vi "Read Regions.vi"(8 "error in (no error)":errorcluster, 11 "SOL Camera in":refnum<class "PL SOL Instruments Camera.lvclass">) -> (0 "error out":errorcluster, 2 "regions":T1(array[cluster]), 3 "SOL Camera out":refnum<class "PL SOL Instruments Camera.lvclass">)   [LabVIEW 2015, in "PL SOL Instruments Camera.lvclass"]
doc: "Reads acquisition regions."
uses:
  PL SOL Instruments Camera.lvclass
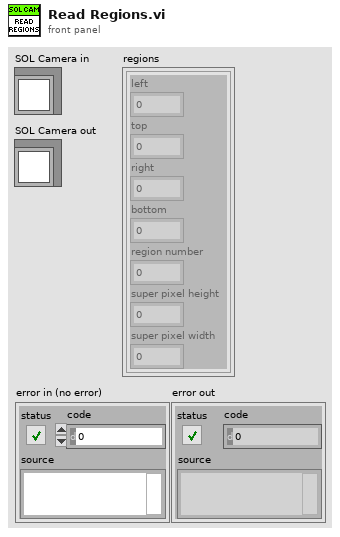
[diagram p1: front panel]
types:
  T1 = cluster{"left":u16, "top":u16, "right":u16, "bottom":u16, "region number":u16, "super pixel height":u16, "super pixel width":u16}[]
  T2 = cluster{"wLeft":u16, "wTop":u16, "wRight":u16, "wBottom":u16, "wRegionNumber":u16, "wSUPixelHeight":u16, "wSUPixelWidth":u16}[]
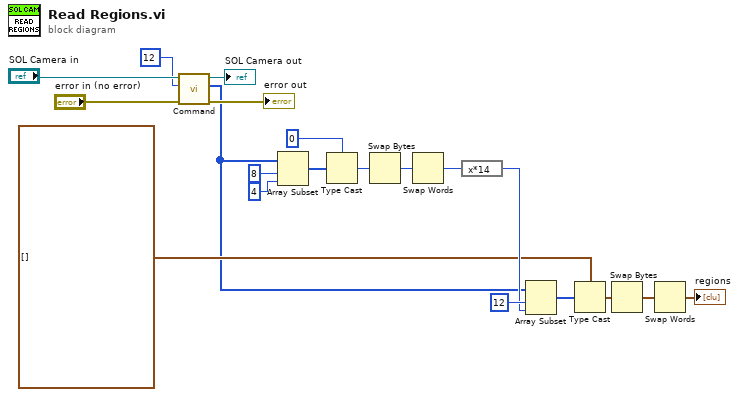
[diagram p0: block diagram]
diagram:
  n1 = call "Command.vi"("error in (no error)"="error in (no error)", "command"=u8 12, "SOL Camera in"="SOL Camera in") -> ("error out"=→"error out":errorcluster, "response"=w2:u8[], "SOL Camera out"=→"SOL Camera out":refnum<class "PL SOL Instruments Camera.lvclass">)  [unwired: 6 in]
  n2 = Array Subset(array=w2, index=8, length=4) -> (w14:u8[])
  n3 = Type Cast(type=u32 0, x=w14) -> (*(type *) &x=w9:u32)
  n4 = Swap Bytes(anything=w9) -> (byte swapped=w10:u32)
  n5 = Swap Words(1:w10) -> (0:w8:u32)
  n6 = expression code="x*14"(w8) -> (w7:u32)
  n7 = Array Subset(array=w2, index=12, length=w7) -> (w13:u8[])
  n8 = Type Cast(type=T2 [], x=w13) -> (*(type *) &x=w4:T2)
  n9 = Swap Bytes(anything=w4) -> (byte swapped=w5:T2)
  n10 = Swap Words(1:w5) -> (0:→"regions":T2)
